vi "Stack PID Fan by Ref.vi"(6 "Reinitialize":bool, 8 "error in":errorcluster, 10 "Temperature":dbl, 11 "PID Ref":refnum<vi>) -> (0 "error out":errorcluster, 3 "Output":u8)   [LabVIEW 2024]
uses:
  <vilib>/addons/control/pid/NI_PID_pid.lvlib
  <vilib>/addons/control/pid/pid.llb/PID (DBL).vi
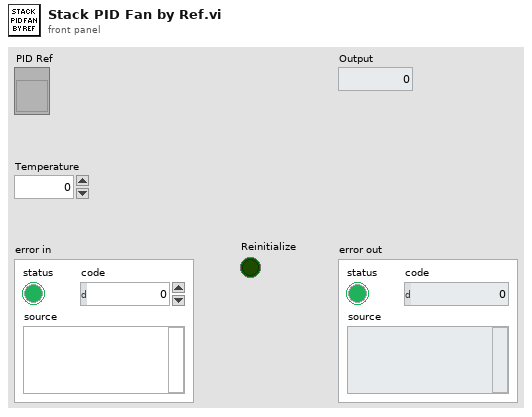
[diagram p1: front panel]
types:
  T1 = cluster{"proportional gain (Kc)":dbl, "integral time (Ti, min)":dbl, "derivative time (Td, min)":dbl}
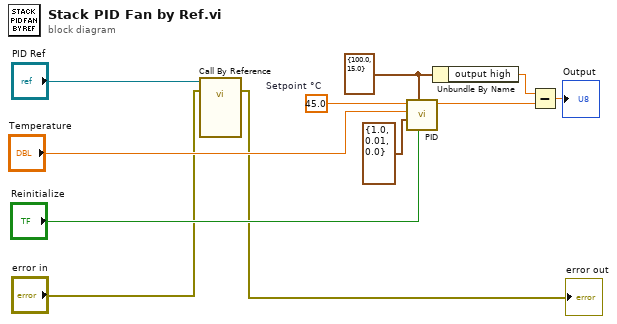
[diagram p0: block diagram]
diagram:
  w10 = 45.0  # Setpoint °C
  w9 = cluster{"output high":dbl, "output low":dbl} {"output high"=100.0, "output low"=15.0} ("output range")
  n1 = call-by-ref "?"(reference="PID Ref", error in="error in") -> (error out=→"error out":errorcluster)  [unwired: 10 in, 3 out]
  n2 = call-poly <vilib>:"PID.vi"("reinitialize? (F)"="Reinitialize", "output range"=w9, "PID gains"=T1 {"proportional gain (Kc)"=1.0, "integral time (Ti, min)"=0.01, "derivative time (Td, min)"=0.0}, "process variable"="Temperature", "setpoint"=w10) -> ("output"=w11:dbl)  [unwired: 5 in, 1 out]
  n3 = Unbundle By Name(w9) -> ("output high"=w1:dbl)
  n4 = Subtract(x=w1, y=w11) -> (x-y=→"Output":dbl)
